vi "Press_Coeff_Read.vi"(8 "error in (no error)":errorcluster, 11 "BMP208 in":refnum<class "BMP208.lvclass">) -> (0 "error out":errorcluster, 3 "BMP208 out":refnum<class "BMP208.lvclass">)   [LabVIEW 2020, in "BMP208.lvclass"]
uses:
  BMP208.lvclass
  BMP208.lvclass/BMP208.ctl
  Properties/Write PressCoeff.vi
  LINX I2C/LINX I2C.lvclass
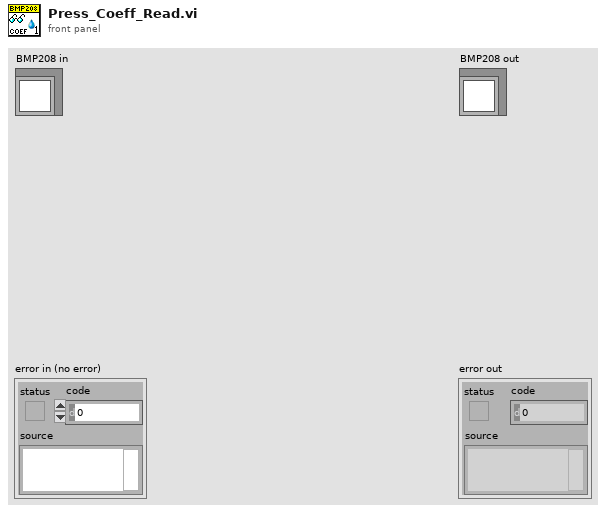
[diagram p1: front panel]
types:
  T1 = cluster{"[0]":u16, "[1]":u16, "[2]":u16, "[3]":u16, "[4]":u16, "[5]":u16, "[6]":u16, "[7]":u16, "[8]":u16}
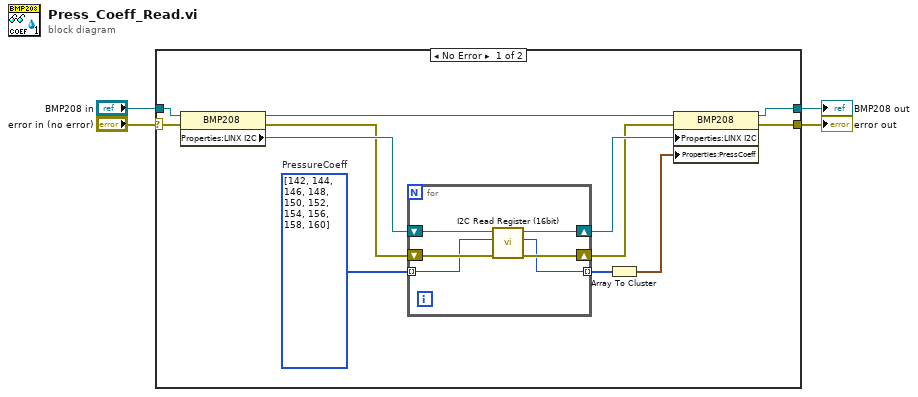
[diagram p0: block diagram]
diagram:
  n1 = case shown="No Error" "error in (no error)" {
    selector: "error in (no error)" -> [w16 w24]
    tunnel: [w14 w24] -> w3
    tunnel: [w12 w23] -> w1
    tunnel: "BMP208 in" -> [w15 w23]
    frame No Error {
      w7 = u8[] [142, 144, 146, 148, 150, 152, 154, 156, 158, 160]  # PressureCoeff
      n2 = property class="BMP208"(reference=w15, error in=w16) -> (reference out=w13:refnum<class "BMP208.lvclass">, error out=w8:errorcluster, "Properties:LINX I2C"=w9:refnum<class "LINX I2C.lvclass">)
      n3 = for {
        shift-right: [w22] -> w11
        shift-left: w9 -> [w20]
        shift-right: [w21] -> w10
        shift-left: w8 -> [w19]
        tunnel: w7 -> [w18] mode=indexing
        tunnel: [w17] -> w6 mode=indexing
        n4 = call "I2C Read Register (16bit).vi"("error in (no error)"=w19, "Register Address"=w18, "LINX I2C in"=w20) -> ("error out"=w21:errorcluster, "Value"=w17:u16, "LINX I2C out"=w22:refnum<class "LINX I2C.lvclass">)  [unwired: 6 in]
      }
      n5 = Array To Cluster(array=w6) -> (cluster=w5:T1)
      n6 = property class="BMP208"(reference=w13, error in=w10, "Properties:LINX I2C"=w11, "Properties:PressCoeff"=w5) -> (reference out=w12:refnum<class "BMP208.lvclass">, error out=w14:errorcluster)
    }
    frame Error {
    }
  }
  "error out" <- w3
  "BMP208 out" <- w1
